vi "GetPhaseDataSets.vi"(10 "Motor Info":T1, 11 "DataSets":T2[](array[typedef])) -> (3 "ValidPhaseDataSets":waveform(sgl)[](array[waveform]))   [LabVIEW 2017, in "McsaStartupAnalysis.lvlib"]
uses:
  <vilib>/addons/InsightCM/Devices/Shared/Mcsa/McsaStartupAnalysis/McsaStartupAnalysis.lvlib
  <vilib>/addons/InsightCM/Devices/Shared/Common/DataEvent/controls/DataSet.ctl
  <vilib>/addons/InsightCM/MessageBus/Base/controls/DataSetMetadata.ctl
  <vilib>/addons/InsightCM/MessageBus/Base/controls/KeyValuePair.ctl
  <vilib>/addons/InsightCM/Devices/Shared/Mcsa/McsaStartupAnalysis/controls/MotorInfo.ctl
  <vilib>/addons/InsightCM/Devices/Shared/Common/DataEvent/DataEvent.lvlib
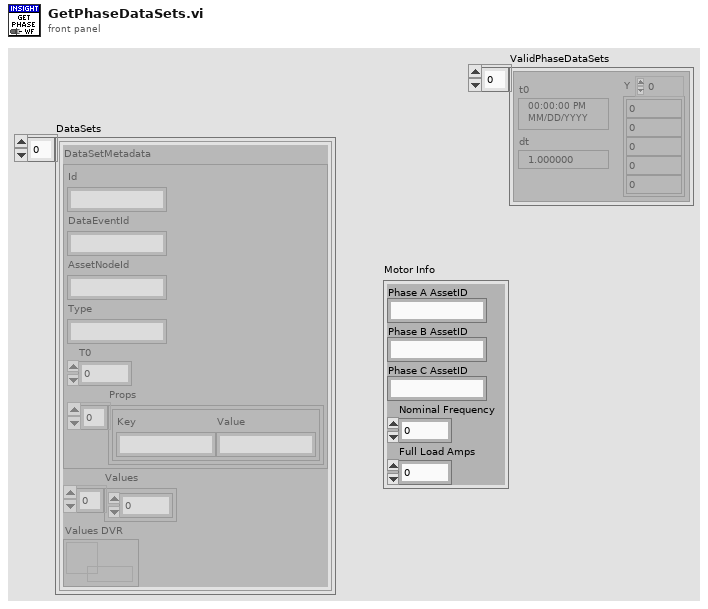
[diagram p1: front panel]
types:
  T1 = typedef "McsaStartupAnalysis.lvlib/MotorInfo.ctl" = cluster{"Phase A AssetID":string, "Phase B AssetID":string, "Phase C AssetID":string, "Nominal Frequency":dbl, "Full Load Amps":dbl}
  T2 = typedef "DataEvent.lvlib/DataSet.ctl" = cluster{"DataSetMetadata":T3, "Values":sgl[], "Values DVR":refnum<data-value>}
  T3 = typedef "DataSetMetadata.ctl" = cluster{"Id":string, "DataEventId":string, "AssetNodeId":string, "Type":string, "T0":i64, "Props":T4[]}
  T4 = typedef "KeyValuePair.ctl" = cluster{"Key":string, "Value":string}
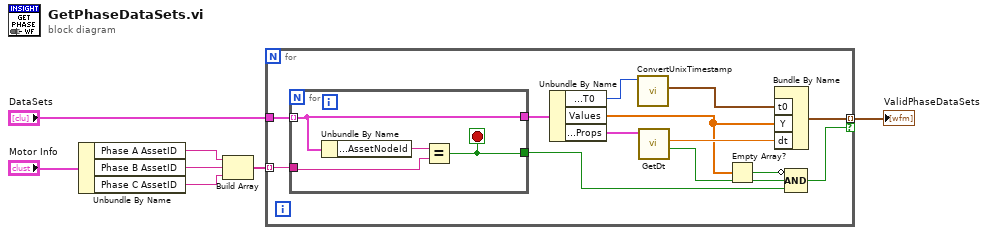
[diagram p0: block diagram]
diagram:
  n1 = Unbundle By Name("Motor Info") -> ("Phase A AssetID"=w5:string, "Phase B AssetID"=w4:string, "Phase C AssetID"=w3:string)
  n2 = Build Array(w5, w4, w3) -> (w2:string[])
  n3 = for {
    tunnel: "DataSets" -> [w20]
    tunnel: w2 -> [w19] mode=indexing
    tunnel: [w13] -> w6 mode=indexing if=w9
    n4 = for {
      tunnel: w20 -> [w22] mode=indexing
      tunnel: w19 -> [w23]
      tunnel: [w22] -> w18
      tunnel: [w21] -> w12
      stop <- w21 stop-if-true
      n5 = Unbundle By Name(w22) -> ("DataSetMetadata.AssetNodeId"=w24:string)
      n6 = Equal?(x=w24, y=w23) -> (x = y?=w21:bool)
    }
    n7 = Unbundle By Name(w18) -> ("DataSetMetadata.T0"=w16:i64, "Values"=w11:sgl[], "DataSetMetadata.Props"=w17:T4[])
    n8 = call <vilib>:"ConvertUnixTimestamp.vi"("Timestamp in"=w16) -> ("Time Stamp out"=w15:timestamp)  [unwired: 10 in]
    n9 = call <vilib>:"GetDt.vi"("props in"=w17) -> ("found"=w8:bool, "Dt"=w14:dbl)  [unwired: 8 in, 1 out]
    n10 = Empty Array?(array=w11) -> (empty?=w10:bool)
    n11 = Bundle By Name("t0"=w15, "Y"=w11, "dt"=w14) -> (w13:waveform(sgl))  [unwired: 1 in]
    n12 = Compound Arithmetic op=AND(invert w10, w8, w12) -> (w9:bool)
  }
  "ValidPhaseDataSets" <- w6
